vi "Engine Out - Faults - Turbo Inlet Air Temp.vi"(11 "Turbo Inlet Air Temp [C]":sgl) -> ()   [LabVIEW 2015, in "ECS-RT.lvlib"]
uses:
  ECS-RT.lvlib
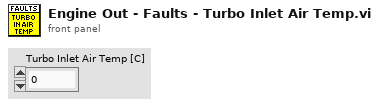
[diagram p1: front panel]
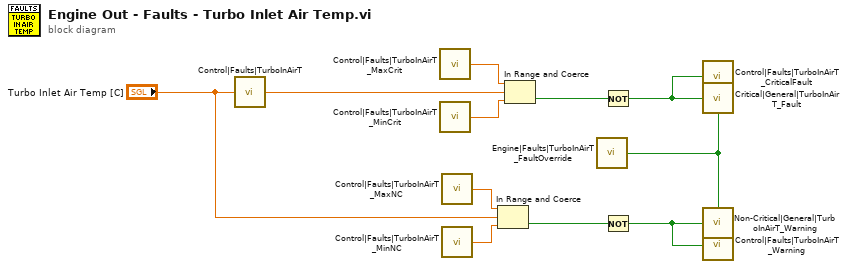
[diagram p0: block diagram]
diagram:
  n1 = call "Control|Faults|TurboInAirT"("Value"="Turbo Inlet Air Temp [C]") -> ()
  n2 = call "Control|Faults|TurboInAirT_MaxCrit"() -> ("Value"=w5:sgl)
  n3 = call "Control|Faults|TurboInAirT_MinCrit"() -> ("Value"=w4:sgl)
  n4 = call "Control|Faults|TurboInAirT_MaxNC"() -> ("Value"=w9:sgl)
  n5 = call "Control|Faults|TurboInAirT_MinNC"() -> ("Value"=w8:sgl)
  n6 = In Range and Coerce(upper limit=w9, x="Turbo Inlet Air Temp [C]", lower limit=w8) -> (In Range?=w7:bool)  [unwired: 1 out]
  n7 = In Range and Coerce(upper limit=w5, x="Turbo Inlet Air Temp [C]", lower limit=w4) -> (In Range?=w3:bool)  [unwired: 1 out]
  n8 = call "Engine|Faults|TurboInAirT_FaultOverride"() -> ("Value"=w1:bool)
  n9 = Not(x=w3) -> (.not. x?=w6:bool)
  n10 = Not(x=w7) -> (.not. x?=w10:bool)
  n11 = call "Control|Faults|TurboInAirT_CriticalFault"("Value"=w6) -> ()
  n12 = call "Critical|General|TurboInAirT_Fault"("Fault"=w6, "Override (F)"=w1) -> ()  [unwired: 1 in]
  n13 = call "Non-Critical|General|TurboInAirT_Warning"("Fault"=w10, "Override (F)"=w1) -> ()  [unwired: 1 in]
  n14 = call "Control|Faults|TurboInAirT_Warning"("Value"=w10) -> ()
